vi "GetRunningServerInfo.vi"(0 "New Server":T2={"vi name"="", "VI Refnum"=refnum, "queue"=refnum, "ROS"={"topic port"=0, "Node"="", "topic"="", "type"="", "node port"=0, "error "={"status"=FALSE, "code"=0, "source"=""}, "Direction"=enum."Node", "APIs"=[], "Update (ms)"=1, "write queue"=1}, "notifier"=refnum}, 1 "Task":T1(ring)=enum."Get Info") -> (2 "Status":T5[](array[typedef]), 3 "servers":T2[](array[typedef]), 4 "Topics":string[](array[string]))   [LabVIEW 2012]
uses:
  <userlib>/ROSforLV/ROS/Code/Console/Servers/ServerSubs/MyState.ctl
  <userlib>/ROSforLV/ROS/Code/Console/Servers/ServerSubs/ServoInfo.ctl
  <userlib>/ROSforLV/ROS/Code/SubVIs/_ROSControl.ctl
  <userlib>/ROSforLV/ROS/Code/SubVIs/_ROSDirection.ctl
panel:
  out "error out":errorcluster
  out "Setups":string[](array[string])
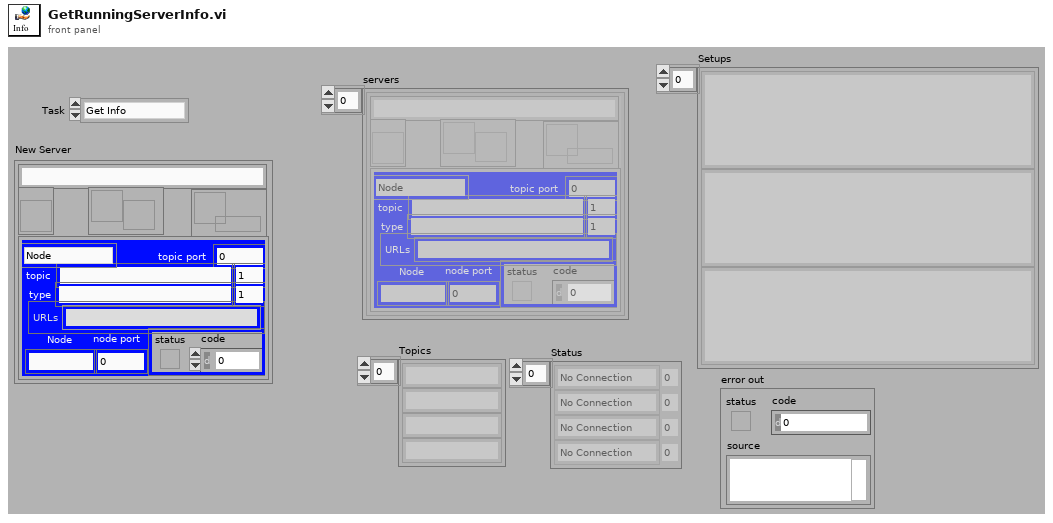
[diagram p1: front panel]
types:
  T1 = enum16{"Add Server", "Clear Server", "Clear All", "Get Info", "GetPanelInfo"}
  T2 = typedef "ServoInfo.ctl" = cluster{"vi name":string, "VI Refnum":refnum<vi>, "queue":refnum<queue>, "ROS":T3, "notifier":refnum<notifier>}
  T3 = typedef "_ROSControl.ctl" = cluster{"topic port":u16, "Node":string, "topic":string, "type":string, "node port":u32, "error ":errorcluster, "Direction":T4, "APIs":string[], "Update (ms)":u16, "write queue":u16}
  T4 = typedef "_ROSDirection.ctl" = enum16{"Node", "Publisher", "Subscriber", "Service Client"}
  T5 = typedef "MyState.ctl" = enum16{"No Connection", "Registered", "Connected", "Close"}
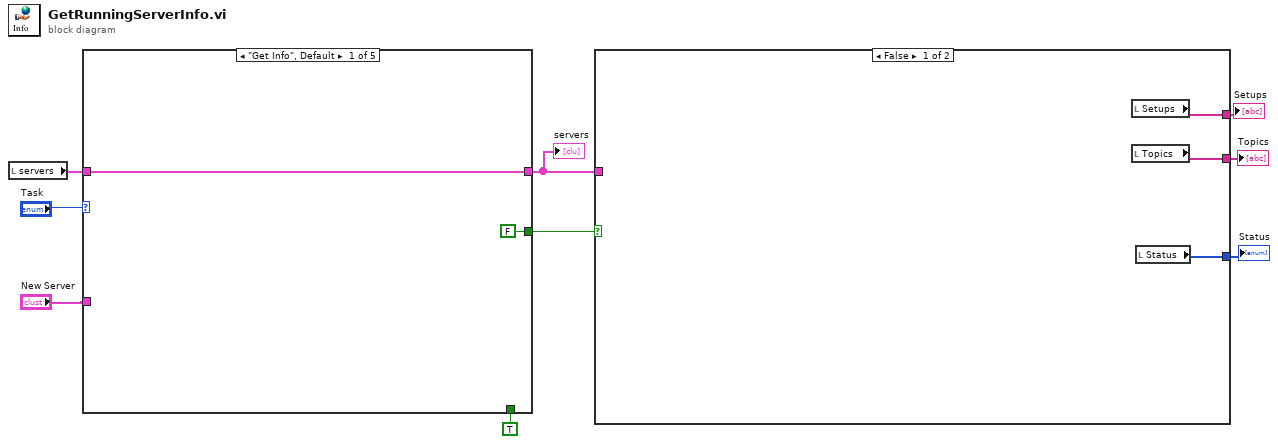
[diagram p0: block diagram]
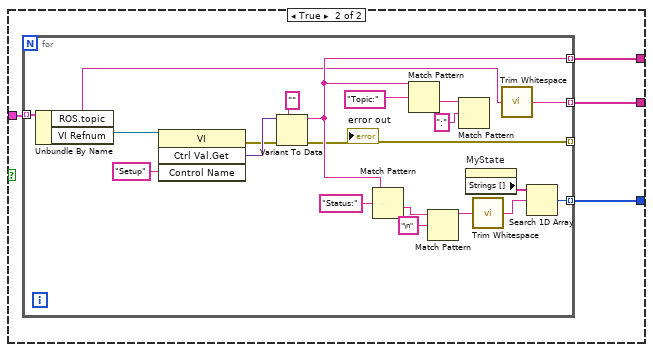
[diagram p2: hidden frame]
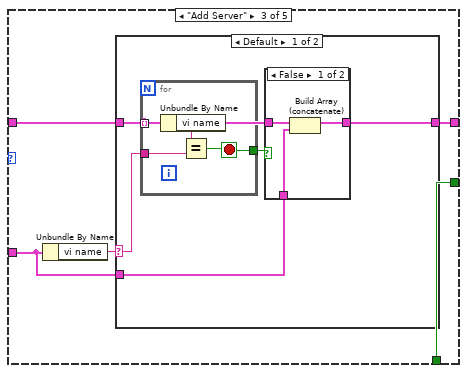
[diagram p4: hidden frame]
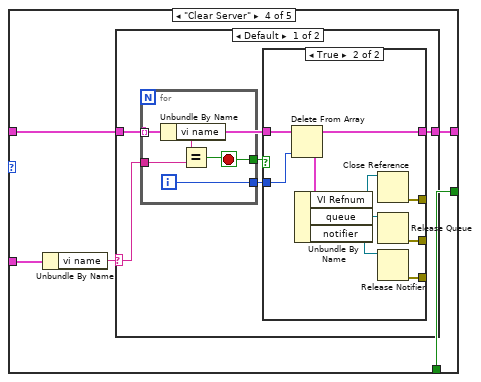
[diagram p7: hidden frame]
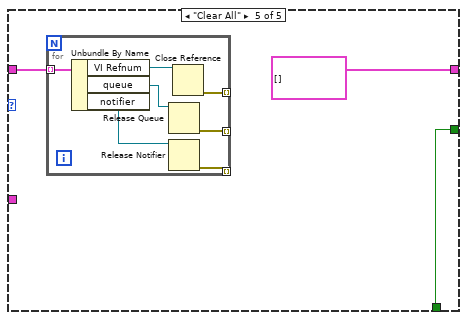
[diagram p10: hidden frame]
diagram:
  n1 = local read "servers"() -> (w2:T2[])
  n2 = case shown="\"Get Info\", Default" "Task" {
    tunnel: w2 -> [w11 w13 w17 w36 w62]
    tunnel: "New Server" -> [_ _ w15 w34 _]
    tunnel: [w11 w13 w16 w35 T2[] [] ("servers")] -> w1
    tunnel: [FALSE ("First Call?: T/F") w12 w14 w33 w61] -> w7
    tunnel: TRUE ("First Call?: T/F") -> [_ w12 w14 w33 w61]
    frame "Get Info", Default {
    }
    frame "GetPanelInfo" {
    }
    frame "Add Server" {
      n3 = Unbundle By Name(w15) -> ("vi name"=w18:string)
      n4 = case shown="Default" w18 {
        selector: w18 -> [w23 _]
        tunnel: [w21 w32] -> w16
        tunnel: w17 -> [w20 w32]
        tunnel: w15 -> [w19 _]
        frame Default {
          n5 = for {
            tunnel: w20 -> [w31] mode=indexing
            tunnel: w23 -> [w29]
            tunnel: [w28] -> w22
            stop <- w28 stop-if-true
            n6 = Unbundle By Name(w31) -> ("vi name"=w30:string)
            n7 = Equal?(x=w30, y=w29) -> (x = y?=w28:bool)
          }
          n8 = case shown="False" w22 {
            tunnel: [w24 w27] -> w21
            tunnel: w20 -> [w26 w27]
            tunnel: w19 -> [w25 _]
            frame False {
              n9 = Build Array (concatenate)(w26, w25) -> (w24:T2[])
            }
            frame True {
            }
          }
        }
        frame "" {
        }
      }
    }
    frame "Clear Server" {
      n10 = Unbundle By Name(w34) -> ("vi name"=w37:string)
      n11 = case shown="Default" w37 {
        selector: w37 -> [w42 _]
        tunnel: [w40 w59] -> w35
        tunnel: w36 -> [w39 w59]
        frame Default {
          n12 = for {
            tunnel: w39 -> [w58] mode=indexing
            tunnel: w42 -> [w56]
            tunnel: [w55] -> w41
            tunnel: [w54] -> w38
            i -> [w54]
            stop <- w55 stop-if-true
            n13 = Unbundle By Name(w58) -> ("vi name"=w57:string)
            n14 = Equal?(x=w57, y=w56) -> (x = y?=w55:bool)
          }
          n15 = case shown="True" w41 {
            tunnel: [w43 w51] -> w40
            tunnel: w39 -> [w43 w52]
            tunnel: w38 -> [_ w53]
            tunnel: [_ w46] -> _
            tunnel: [_ w45] -> _
            tunnel: [_ w44] -> _
            frame False {
            }
            frame True {
              n16 = Delete From Array(array=w52, index=w53) -> (deleted portion=w50:T2, array with subset deleted=w51:T2[])  [unwired: 1 in]
              n17 = Unbundle By Name(w50) -> ("VI Refnum"=w47:refnum<vi>, "queue"=w49:refnum<queue>, "notifier"=w48:refnum<notifier>)
              n18 = Close Reference(reference=w47) -> (error out=w46:errorcluster)  [unwired: 1 in]
              n19 = Release Queue(queue=w49) -> (error out=w45:errorcluster)  [unwired: 2 in, 2 out]
              n20 = Release Notifier(notifier=w48) -> (error out=w44:errorcluster)  [unwired: 2 in, 2 out]
            }
          }
        }
        frame "" {
        }
      }
    }
    frame "Clear All" {
      n21 = for {
        tunnel: w62 -> [w69] mode=indexing
        tunnel: [w67] -> _ mode=indexing
        tunnel: [w64] -> _ mode=indexing
        tunnel: [w63] -> _ mode=indexing
        n22 = Unbundle By Name(w69) -> ("VI Refnum"=w68:refnum<vi>, "queue"=w66:refnum<queue>, "notifier"=w65:refnum<notifier>)
        n23 = Release Queue(queue=w66) -> (error out=w64:errorcluster)  [unwired: 2 in, 2 out]
        n24 = Release Notifier(notifier=w65) -> (error out=w63:errorcluster)  [unwired: 2 in, 2 out]
        n25 = Close Reference(reference=w68) -> (error out=w67:errorcluster)  [unwired: 1 in]
      }
    }
  }
  "servers" <- w1
  n26 = case shown="False" w7 {
    tunnel: w1 -> [_ w76]
    tunnel: [w71 w75] -> w5
    tunnel: [w70 w74] -> w4
    tunnel: [w72 w73] -> w3
    frame False {
      n27 = local read "Setups"() -> (w71:string[])
      n28 = local read "Topics"() -> (w70:string[])
      n29 = local read "Status"() -> (w72:T5[])
    }
    frame True {
      n30 = for {
        tunnel: w76 -> [w82] mode=indexing
        tunnel: [w93] -> w74 mode=indexing
        tunnel: [w86] -> w73 mode=indexing
        tunnel: [w78] -> _ mode=indexing
        tunnel: [w80] -> w75 mode=indexing
        n31 = Unbundle By Name(w82) -> ("ROS.topic"=w77:string, "VI Refnum"=w81:refnum<vi>)
        n32 = invoke class="VI" method="Ctrl Val.Get"(reference=w81, "Control Name"="Setup") -> (error out=w79:errorcluster, "Get Control Value Variant"=w84:variant)  [unwired: 2 in, 2 out]
        n33 = Variant To Data(error in=w79, type="" ("Control Name"), Variant=w84) -> (data=w80:string, error out=w78:errorcluster)
        "error out" <- w78
        n34 = Match Pattern(string=w80, regular expression="Status:") -> (after substring=w91:string)  [unwired: 1 in, 3 out]
        n35 = Match Pattern(string=w80, regular expression="Topic:") -> (after substring=w95:string)  [unwired: 1 in, 3 out]
        n36 = Match Pattern(string=w91, regular expression="\n") -> (before substring=w89:string)  [unwired: 1 in, 3 out]
        n37 = Match Pattern(string=w95, regular expression=":") -> ()  [unwired: 1 in, 4 out]
        n38 = property on="MyState" class="Enum (strict)"() -> ("Strings []"=w88:string[])  [unwired: 2 in, 2 out]
        n39 = call <vilib>:"Trim Whitespace.vi"("string"=w89) -> ("trimmed string"=w87:string)  [unwired: 1 in]
        n40 = call <vilib>:"Trim Whitespace.vi"("string"=w77) -> ("trimmed string"=w93:string)  [unwired: 1 in]
        n41 = Search 1D Array(1D array=w88, element=w87) -> (index of element=w86:i32)  [unwired: 1 in]
      }
    }
  }
  "Topics" <- w4
  "Status" <- w3
  "Setups" <- w5
